vi "Dialog_Enter Stage Position.vi"(8 "Error In":errorcluster) -> (0 "Error Out":errorcluster, 2 "Cancelled?":bool, 3 "Macro Command":string)   [LabVIEW 2012]
doc: "SciScan 1.2 160622"
uses:
  Custom Controls/Stage Position Data.ctl
  GFG/GFG library.lvlib
panel:
  in  "Update Current Position":bool
  in  "Stage Position Data":T1 caption="Stage Position"
  in  "Cancel Button":bool
  in  "OK Button":bool
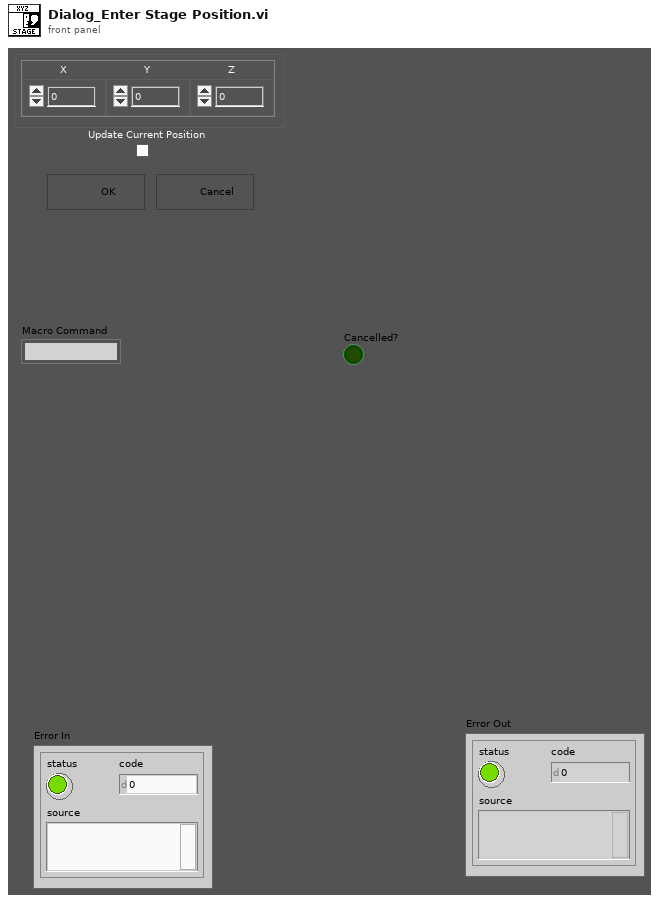
[diagram p1: front panel]
types:
  T1 = typedef "Stage Position Data.ctl" = cluster{"X":dbl, "Y":dbl, "Z":dbl}
  T2 = enum8{"Enabled", "Disabled", "Disabled and Grayed Out"}
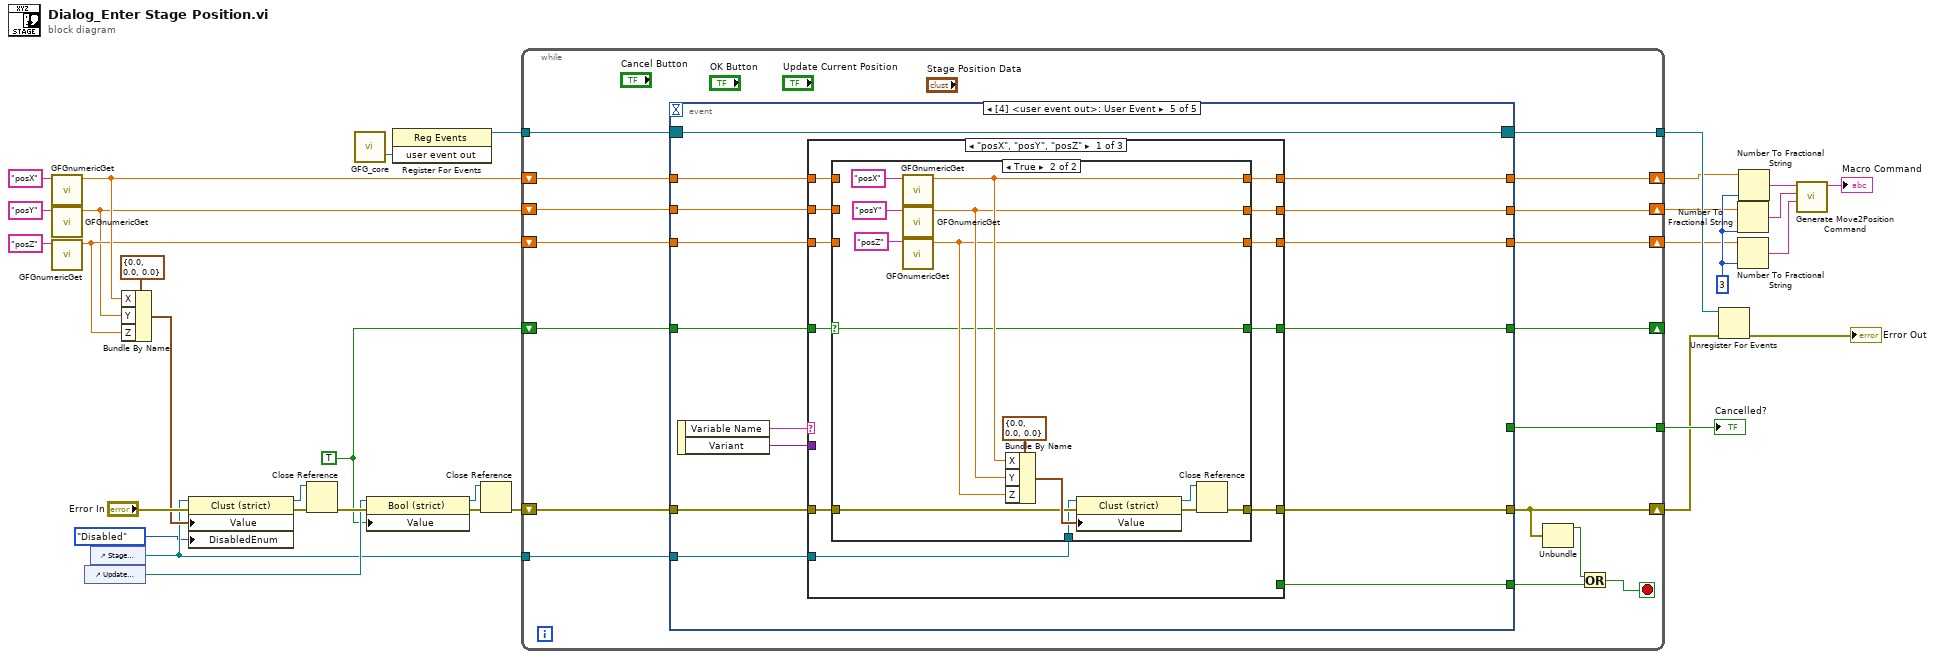
[diagram p0: block diagram]
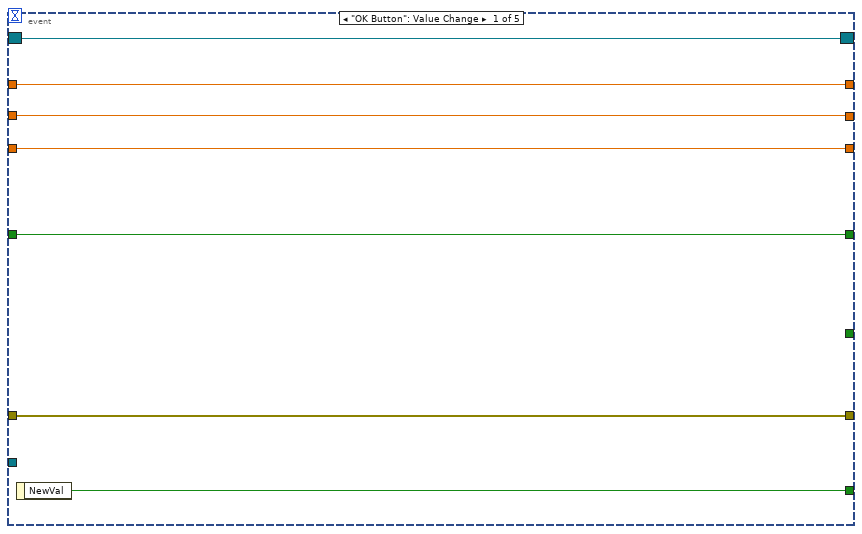
[diagram p2: hidden frame]
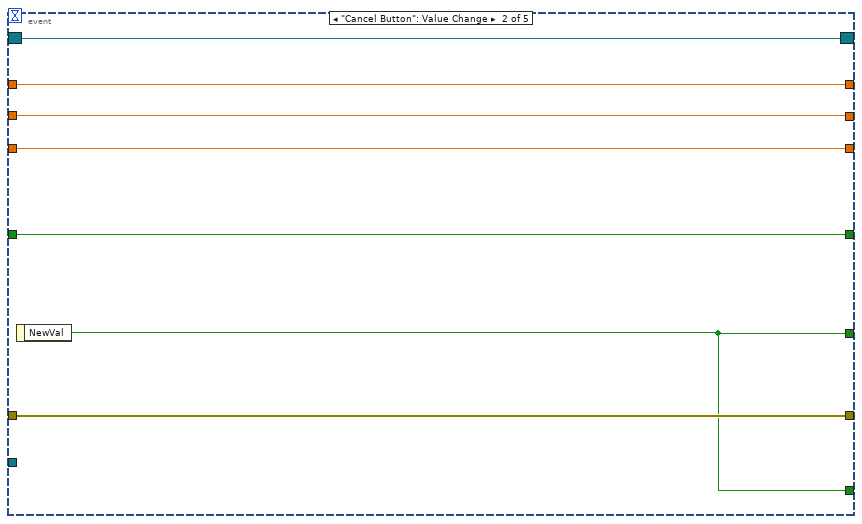
[diagram p3: hidden frame]
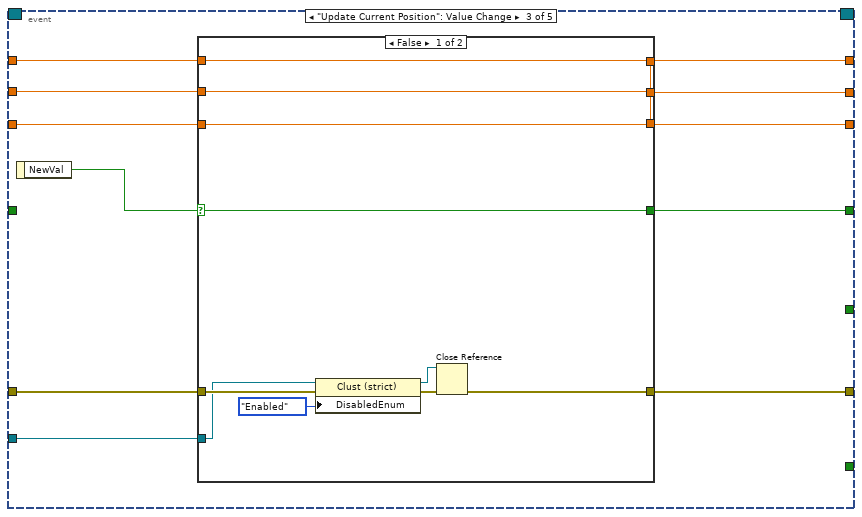
[diagram p4: hidden frame]
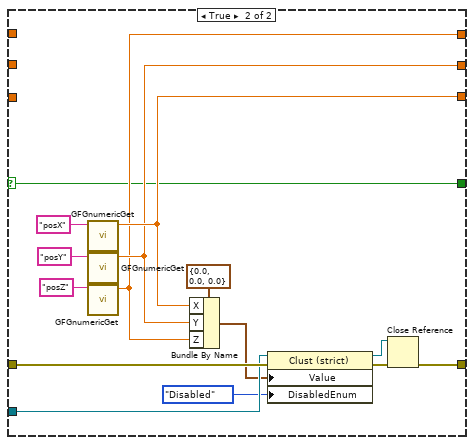
[diagram p5: hidden frame]
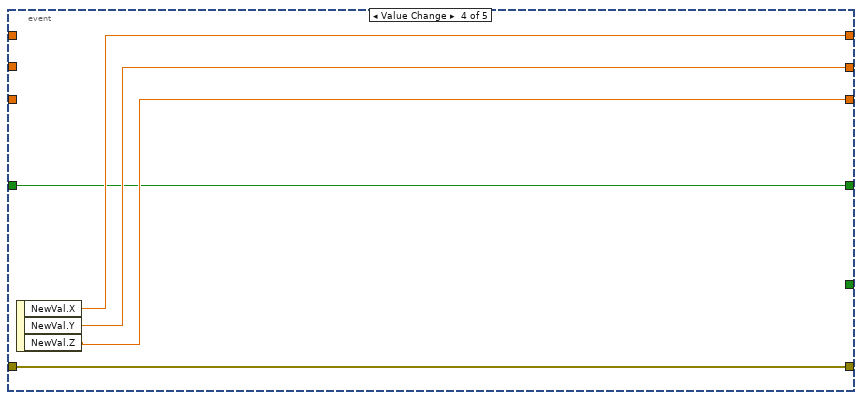
[diagram p6: hidden frame]
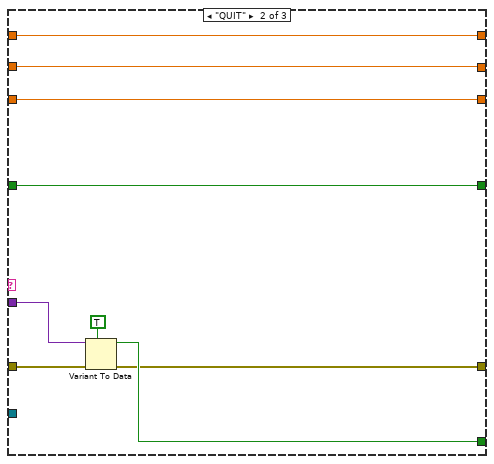
[diagram p8: hidden frame]
diagram:
  w4 = TRUE
  w24 = i16 3 ("precision (6)")
  n1 = call "GFGnumericGet.vi"("Variable Name in"="posX") -> ("Numeric"=w12:dbl)  [unwired: 8 in, 2 out]
  n2 = call "GFGnumericGet.vi"("Variable Name in"="posY") -> ("Numeric"=w10:dbl)  [unwired: 8 in, 2 out]
  n3 = call "GFGnumericGet.vi"("Variable Name in"="posZ") -> ("Numeric"=w11:dbl)  [unwired: 8 in, 2 out]
  n4 = control-ref of="Update Current Position"() -> (w5:refnum<vi>)
  n5 = control-ref of="Stage Position Data"() -> (w2:refnum<vi>)
  n6 = Bundle By Name(cluster=T1 {"X"=0.0, "Y"=0.0, "Z"=0.0} ("Value"), "X"=w12, "Y"=w10, "Z"=w11) -> (w9:T1)
  n7 = property class="Clust (strict)"(reference=w2, error in="Error In", "Value"=w9, "DisabledEnum"=T2."Disabled" ("Disabled")) -> (reference out=w25:refnum<vi>, error out=w26:errorcluster)
  n8 = Close Reference(reference=w25, error in (no error)=w26) -> (error out=w6:errorcluster)
  n9 = call "GFG_core.vi"() -> ("user event out"=w33:refnum<user-event>)  [unwired: 13 in, 6 out]
  n10 = property class="Bool (strict)"(reference=w5, error in=w6, "Value"=w4) -> (reference out=w8:refnum<vi>, error out=w7:errorcluster)
  n11 = register-events(w33) -> (reference out=w32:refnum<event-registration>)  [unwired: 2 in, 1 out]
  n12 = Close Reference(reference=w8, error in (no error)=w7) -> (error out=w3:errorcluster)
  n13 = while {
    tunnel: w32 -> [w50]
    tunnel: [w49] -> w31
    tunnel: [w48] -> w30
    shift-right: [w47] -> w28
    shift-left: w3 -> [w43]
    shift-right: [w40] -> w17
    shift-left: w11 -> [w37]
    shift-right: [w41] -> w18
    shift-left: w10 -> [w38]
    shift-right: [w42] -> w19
    shift-left: w12 -> [w39]
    shift-right: [w36] -> _
    shift-left: w4 -> [w35]
    tunnel: w2 -> [w34]
    stop <- w44 stop-if-true
    n14 = event shown="[4] <user event out>: User Event" {
      selector: w50 -> [w57 w64 _ _ w117]
      dyn-events: [w57 w64 _ _ w117] -> w49
      timeout: _ -> [_ _ _ _ _]
      tunnel: [w52 w62 _ _ w118] -> w46
      tunnel: [_ w62 _ _ _] -> w48
      tunnel: w43 -> [w56 w63 w75 w105 w110]
      tunnel: [w56 w63 w74 w105 w108] -> w47
      tunnel: [w55 w61 w73 w104 w113] -> w42
      tunnel: [w54 w60 w72 w103 w112] -> w41
      tunnel: [w53 w59 w71 w102 w111] -> w40
      tunnel: w39 -> [w55 w61 w68 _ w116]
      tunnel: w38 -> [w54 w60 w67 _ w115]
      tunnel: w37 -> [w53 w59 w66 _ w114]
      tunnel: [w51 w58 w69 w101 w106] -> w36
      tunnel: w35 -> [w51 w58 _ w101 w107]
      tunnel: w34 -> [_ _ w65 _ w109]
      event "OK Button": Value Change {
        n15 = event-data() -> ("NewVal"=w52:bool)  [unwired: 1 in]
      }
      event "Cancel Button": Value Change {
        n16 = event-data() -> ("NewVal"=w62:bool)  [unwired: 1 in]
      }
      event "Update Current Position": Value Change {
        n17 = event-data() -> ("NewVal"=w70:bool)  [unwired: 1 in]
        n18 = case shown="False" w70 {
          selector: w70 -> [w85 w87]
          tunnel: w75 -> [w81 w100]
          tunnel: [w76 w99] -> w74
          tunnel: w65 -> [w80 w93]
          tunnel: [w84 w90] -> w73
          tunnel: [w83 w89] -> w72
          tunnel: [w82 w88] -> w71
          tunnel: [w85 w87] -> w69
          tunnel: w68 -> [w82 _]
          tunnel: w67 -> [w83 _]
          tunnel: w66 -> [w84 _]
          frame False {
            n19 = property class="Clust (strict)"(reference=w80, error in=w81, "DisabledEnum"=T2."Enabled" ("Disabled")) -> (reference out=w77:refnum<vi>, error out=w78:errorcluster)
            n20 = Close Reference(reference=w77, error in (no error)=w78) -> (error out=w76:errorcluster)
          }
          frame True {
            n21 = call "GFGnumericGet.vi"("Variable Name in"="posX") -> ("Numeric"=w90:dbl)  [unwired: 8 in, 2 out]
            n22 = call "GFGnumericGet.vi"("Variable Name in"="posY") -> ("Numeric"=w89:dbl)  [unwired: 8 in, 2 out]
            n23 = call "GFGnumericGet.vi"("Variable Name in"="posZ") -> ("Numeric"=w88:dbl)  [unwired: 8 in, 2 out]
            n24 = Bundle By Name(cluster=T1 {"X"=0.0, "Y"=0.0, "Z"=0.0} ("Stage Position Data"), "X"=w90, "Y"=w89, "Z"=w88) -> (w91:T1)
            n25 = property class="Clust (strict)"(reference=w93, error in=w100, "Value"=w91, "DisabledEnum"=T2."Disabled" ("Disabled")) -> (reference out=w95:refnum<vi>, error out=w94:errorcluster)
            n26 = Close Reference(reference=w95, error in (no error)=w94) -> (error out=w99:errorcluster)
          }
        }
      }
      event Value Change {
        n27 = event-data() -> ("NewVal.X"=w104:dbl, "NewVal.Y"=w103:dbl, "NewVal.Z"=w102:dbl)  [unwired: 1 in]
      }
      event User Event {
        n28 = event-data() -> ("Variable Name"=w120:string, "Variant"=w119:variant)  [unwired: 1 in]
        n29 = case shown="\"posX\", \"posY\", \"posZ\"" w120 {
          tunnel: w119 -> [_ w158 _]
          tunnel: [_ w157 _] -> w118
          tunnel: w116 -> [w121 w156 w164]
          tunnel: w115 -> [w122 w155 w163]
          tunnel: w114 -> [w123 w154 w162]
          tunnel: [w130 w156 w164] -> w113
          tunnel: [w129 w155 w163] -> w112
          tunnel: [w128 w154 w162] -> w111
          tunnel: w110 -> [w131 w153 w161]
          tunnel: w109 -> [w127 _ _]
          tunnel: [w126 w152 w161] -> w108
          tunnel: w107 -> [w125 w151 w160]
          tunnel: [w124 w151 w160] -> w106
          frame "posX", "posY", "posZ" {
            n30 = case shown="True" w125 {
              selector: w125 -> [w136 w137]
              tunnel: w131 -> [w135 w143]
              tunnel: [w132 w142] -> w130
              tunnel: [w133 w141] -> w129
              tunnel: [w134 w140] -> w128
              tunnel: w127 -> [_ w139]
              tunnel: [w135 w138] -> w126
              tunnel: [w136 w137] -> w124
              tunnel: w123 -> [w134 _]
              tunnel: w122 -> [w133 _]
              tunnel: w121 -> [w132 _]
              frame False {
              }
              frame True {
                n31 = call "GFGnumericGet.vi"("Variable Name in"="posX") -> ("Numeric"=w142:dbl)  [unwired: 8 in, 2 out]
                n32 = call "GFGnumericGet.vi"("Variable Name in"="posY") -> ("Numeric"=w141:dbl)  [unwired: 8 in, 2 out]
                n33 = call "GFGnumericGet.vi"("Variable Name in"="posZ") -> ("Numeric"=w140:dbl)  [unwired: 8 in, 2 out]
                n34 = Bundle By Name(cluster=T1 {"X"=0.0, "Y"=0.0, "Z"=0.0} ("Stage Position Data"), "X"=w142, "Y"=w141, "Z"=w140) -> (w144:T1)
                n35 = property class="Clust (strict)"(reference=w139, error in=w143, "Value"=w144) -> (reference out=w147:refnum<vi>, error out=w146:errorcluster)
                n36 = Close Reference(reference=w147, error in (no error)=w146) -> (error out=w138:errorcluster)
              }
            }
          }
          frame "QUIT" {
            n37 = Variant To Data(error in=w153, type=TRUE, Variant=w158) -> (data=w157:bool, error out=w152:errorcluster)
          }
          frame Default {
          }
        }
      }
    }
    n38 = Unbundle(w47) -> ("status"=w45:bool)  [unwired: 2 out]
    n39 = Or(x=w45, y=w46) -> (x .or. y?=w44:bool)
  }
  "Cancelled?" <- w30
  n40 = Unregister For Events(event registration refnum=w31, error in=w28) -> (error out=→"Error Out":errorcluster)
  n41 = Number To Fractional String(number=w18, precision (6)=w24) -> (F-format string=w22:string)  [unwired: 2 in]
  n42 = Number To Fractional String(number=w17, precision (6)=w24) -> (F-format string=w21:string)  [unwired: 2 in]
  n43 = Number To Fractional String(number=w19, precision (6)=w24) -> (F-format string=w23:string)  [unwired: 2 in]
  n44 = call "Generate Move2Position Command.vi"("Pos.Z(um)"=w21, "Pos.Y(um)"=w22, "Pos.X(um)"=w23) -> ("Move2Position Command OUT"=→"Macro Command":string)  [unwired: 7 in, 1 out]
